vi "SaveManMeasure.vi"(6 "EN":bool, 7 "Space":T2, 8 "MeasureUp":T1, 9 "MeasureDown":T1, 10 "Measure Name":string(combo)="DL", 11 "MasterPath":path=path "D:/Output") -> (0 "SaveOK":bool, 1 "File path":path, 3 "Folder path":path)   [LabVIEW 2017]
uses:
  <vilib>/Utility/file.llb/Write Delimited Spreadsheet (string).vi
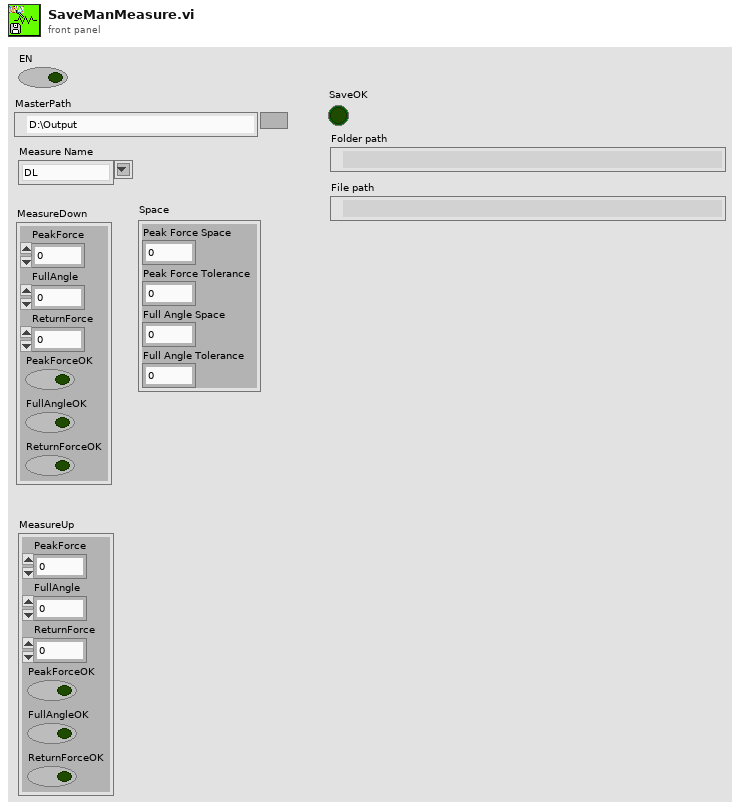
[diagram p1: front panel]
types:
  T1 = cluster{"PeakForce":dbl, "FullAngle":dbl, "ReturnForce":dbl, "PeakForceOK":bool, "FullAngleOK":bool, "ReturnForceOK":bool}
  T2 = cluster{"Peak Force Space":dbl, "Peak Force Tolerance":dbl, "Full Angle Space":dbl, "Full Angle Tolerance":dbl}
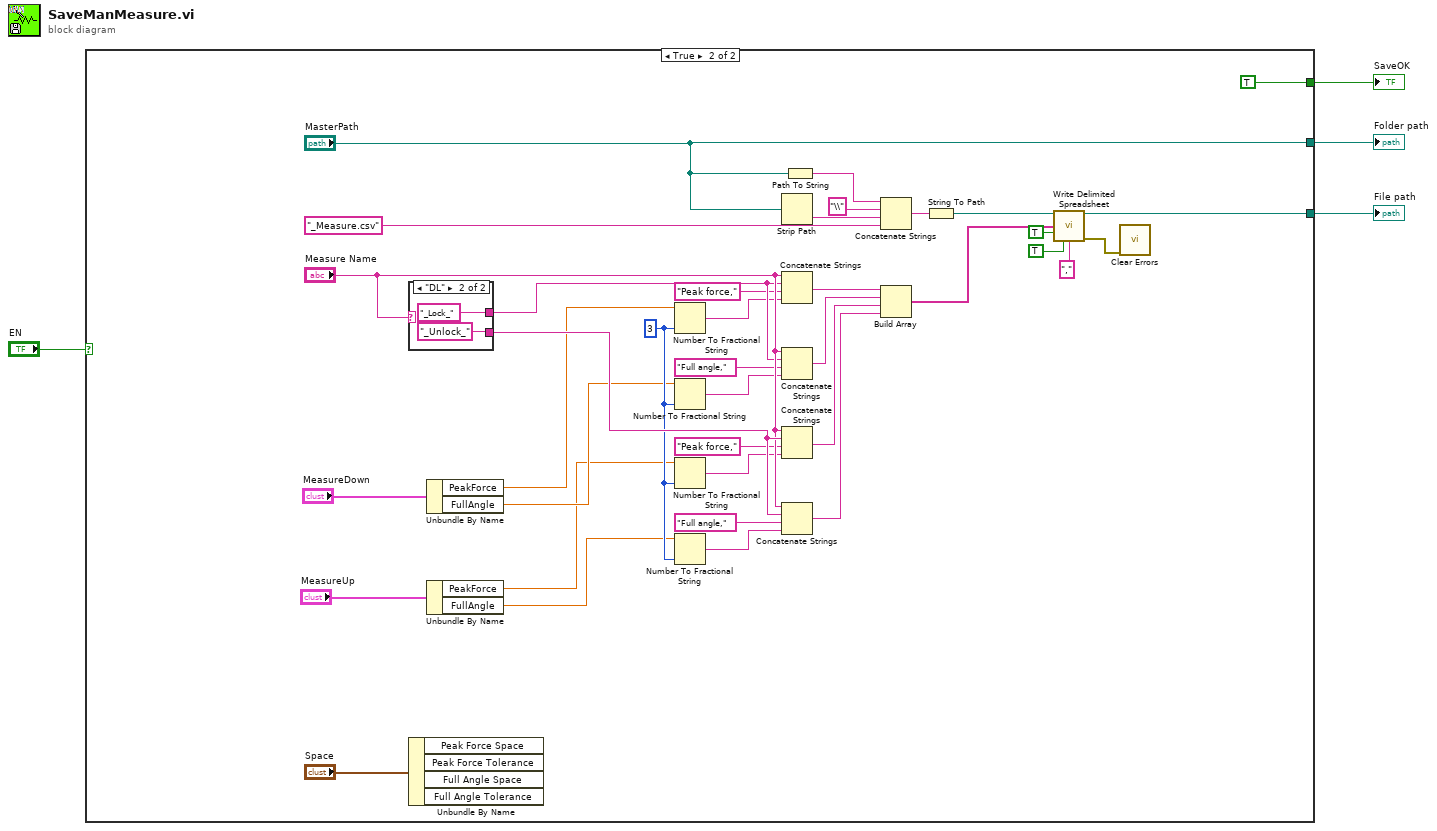
[diagram p0: block diagram]
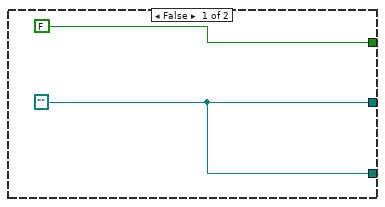
[diagram p2: hidden frame]
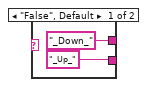
[diagram p3: hidden frame]
diagram:
  n1 = case shown="True" "EN" {
    tunnel: [w5 "MasterPath"] -> w4
    tunnel: [FALSE TRUE] -> w3
    tunnel: [w5 w42] -> w2
    frame False {
      w5 = path ""
    }
    frame True {
      w21 = i16 3 ("precision (6)")
      n2 = case shown="\"DL\"" "Measure Name" {
        tunnel: ["_Down_" ("string") "_Lock_" ("string")] -> w26
        tunnel: ["_Up_" ("string") "_Unlock_" ("string")] -> w31
        frame "False", Default {
        }
        frame "DL" {
        }
      }
      n3 = Unbundle By Name("Space") -> ()  [unwired: 4 out]
      n4 = Unbundle By Name("MeasureDown") -> ("PeakForce"=w22:dbl, "FullAngle"=w10:dbl)
      n5 = Unbundle By Name("MeasureUp") -> ("PeakForce"=w8:dbl, "FullAngle"=w7:dbl)
      n6 = Number To Fractional String(number=w22, precision (6)=w21) -> (F-format string=w23:string)  [unwired: 2 in]
      n7 = Number To Fractional String(number=w10, precision (6)=w21) -> (F-format string=w25:string)  [unwired: 2 in]
      n8 = Number To Fractional String(number=w8, precision (6)=w21) -> (F-format string=w29:string)  [unwired: 2 in]
      n9 = Number To Fractional String(number=w7, precision (6)=w21) -> (F-format string=w28:string)  [unwired: 2 in]
      n10 = Strip Path(path="MasterPath") -> (name=w13:string)  [unwired: 1 out]
      n11 = Concatenate Strings("Measure Name", w26, "Peak force," ("string"), w23) -> (w24:string)
      n12 = Concatenate Strings("Measure Name", w26, "Full angle," ("string"), w25) -> (w27:string)
      n13 = Concatenate Strings("Measure Name", w31, "Peak force," ("string"), w29) -> (w32:string)
      n14 = Concatenate Strings("Measure Name", w31, "Full angle," ("string"), w28) -> (w33:string)
      n15 = Path To String(path="MasterPath") -> (string=w34:string)
      n16 = Concatenate Strings(w34, "\\" ("string"), w13, "_Measure.csv" ("string")) -> (w38:string)
      n17 = Build Array(w24, w27, w32, w33) -> (w16:string[])
      n18 = String To Path(string=w38) -> (path=w37:path)
      n19 = call-poly <vilib>:"Write Delimited Spreadsheet.vi"("file path (dialog if empty)"=w37, "1D data"=w16, "append to file? (new file:F)"=TRUE, "transpose? (no:F)"=TRUE, "delimiter (\\t)"="," ("delimiter (\\t)")) -> ("new file path (Not A Path if cancelled)"=w42:path, "error out"=w36:errorcluster)  [unwired: 9 in]
      n20 = call <vilib>:"Clear Errors.vi"("error in (no error)"=w36) -> ()  [unwired: 5 in, 2 out]
    }
  }
  "Folder path" <- w4
  "SaveOK" <- w3
  "File path" <- w2
